vi "createRedrawCursorsEvent.vi"(8 "error in (no error)":errorcluster, 11 "QControl_Graph in":refnum<class "QControl_Graph.lvclass">) -> (0 "error out":errorcluster, 3 "QControl_Graph out":refnum<class "QControl_Graph.lvclass">)   [LabVIEW 2017, in "QControl_Graph.lvclass"]
uses:
  QControl_Graph.lvclass
  QControl_Graph.lvclass/QControl_Graph.ctl
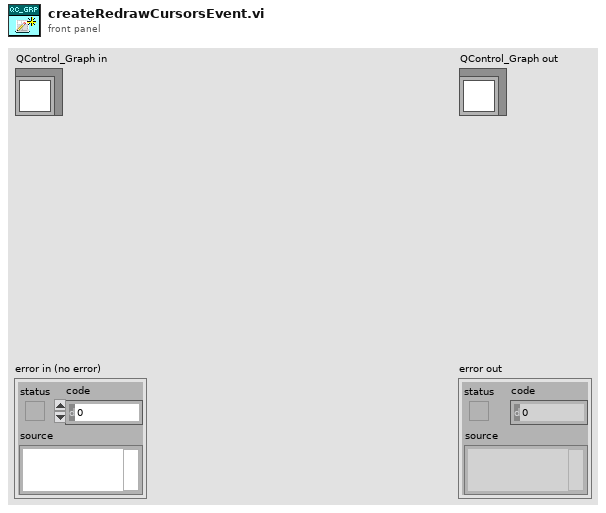
[diagram p1: front panel]
types:
  T1 = typedef "QControl_Graph.lvclass/State Data.ctl" = cluster{"Action Performed":refnum<user-event>, "Show Cursors":bool, "Cursor Properties":T2, "Redraw Cursors":refnum<user-event>}
  T2 = typedef "QControl_Graph.lvclass/Cursor Properties.ctl" = cluster{"Horizontal Line?":bool, "Vertical Line?":bool, "Timestamp":enum16{"at TOP", "at BOTTOM", "none"}, "time format (%H:%M:%S)":string, "size":i16, "font":T3, "alignment(left, top)":T4, "TextFormat":string}
  T3 = typedef "QControl_Graph.lvclass/Font.ctl" = cluster{"Font Name":string, "Size":i16, "Strikeout?":bool, "Italic?":bool, "Underline?":bool, "Outline?":bool, "Shadow":bool, "Bold?":bool}
  T4 = typedef "QControl_Graph.lvclass/Alignment.ctl" = cluster{"Horizontal":T5, "Vertical":T6}
  T5 = typedef "QControl_Graph.lvclass/Alignment.Horizontal.ctl" = enum16{"left", "center", "right"}
  T6 = typedef "QControl_Graph.lvclass/Alignment.Vertical.ctl" = enum16{"top", "center", "bottom"}
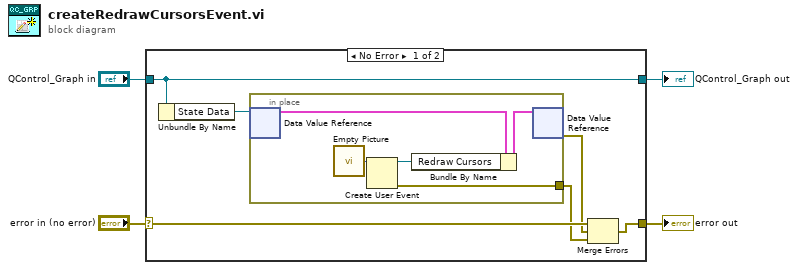
[diagram p0: block diagram]
diagram:
  n1 = case shown="No Error" "error in (no error)" {
    selector: "error in (no error)" -> [w10 w17]
    tunnel: [w7 w17] -> w3
    tunnel: [w9 w16] -> w1
    tunnel: "QControl_Graph in" -> [w9 w16]
    frame No Error {
      n2 = Unbundle By Name(w9) -> ("State Data"=w8:refnum<data-value>)
      n3 = in-place {
        in-place-border: [w15] -> w5
        n4 = in-place-dvr #1(w8) -> (w14:T1)  [unwired: 1 out]
        n5 = call "Empty Picture"() -> ("empty picture"=w11:picture)
        n6 = Create User Event(user event datatype=w11) -> (user event=w12:refnum<user-event>, error out=w15:errorcluster)  [unwired: 1 in]
        n7 = Bundle By Name(cluster=w14, "Redraw Cursors"=w12) -> (w13:T1)
        n8 = in-place-dvr #1(w13) -> (w6:errorcluster)  [unwired: 1 out]
      }
      n9 = Merge Errors(w10, w6, w5) -> (w7:errorcluster)
    }
    frame Error {
    }
  }
  "error out" <- w3
  "QControl_Graph out" <- w1
